vi "Write Filter.vi"(0 "fpga reference in":T2, 2 "enable filter":bool=TRUE, 7 "coefficients":T1, 11 "error in":errorcluster) -> (4 "fpga reference out":T2, 15 "error out":errorcluster)   [LabVIEW 2019]
uses:
  TypeDefs/Blank FPGA Reference.ctl
  <vilib>/rvi/errors/niLvFpgaAdjustHostInterfaceError.vi
  <vilib>/rvi/interface/nirviReadWriteControl/nirviReadWriteControl.xnode
  <vilib>/rvi/interface/Simulation/niFpgaSimulationCallBeginRW.vi
  NiFpgaLv.dll
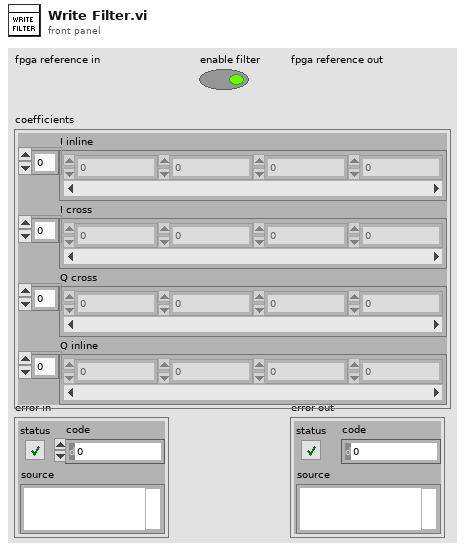
[diagram p1: front panel]
types:
  T1 = cluster{"I inline":dbl[], "I cross":dbl[], "Q cross":dbl[], "Q inline":dbl[]}
  T2 = typedef "Blank FPGA Reference.ctl" = refnum<k20>
  T3 = enum8{"None", "I Inline", "I Cross", "Q Cross", "Q Inline"}
  T4 = cluster{"filter select":enum8{"None", "I Inline", "I Cross", "Q Cross", "Q Inline"}, "coef load":bool, "coef write":bool, "coef data":fxp<+/-,18,1>}
  T5 = enum8{"None", "I Inline", "I Cross", "Q Cross", "Q Inline"}[]
  T6 = cluster{"filter select":enum8{"None", "I Inline", "I Cross", "Q Cross", "Q Inline"}, "coef load":bool, "coef write":bool, "coef data":fxp<+/-,18,1>}[]
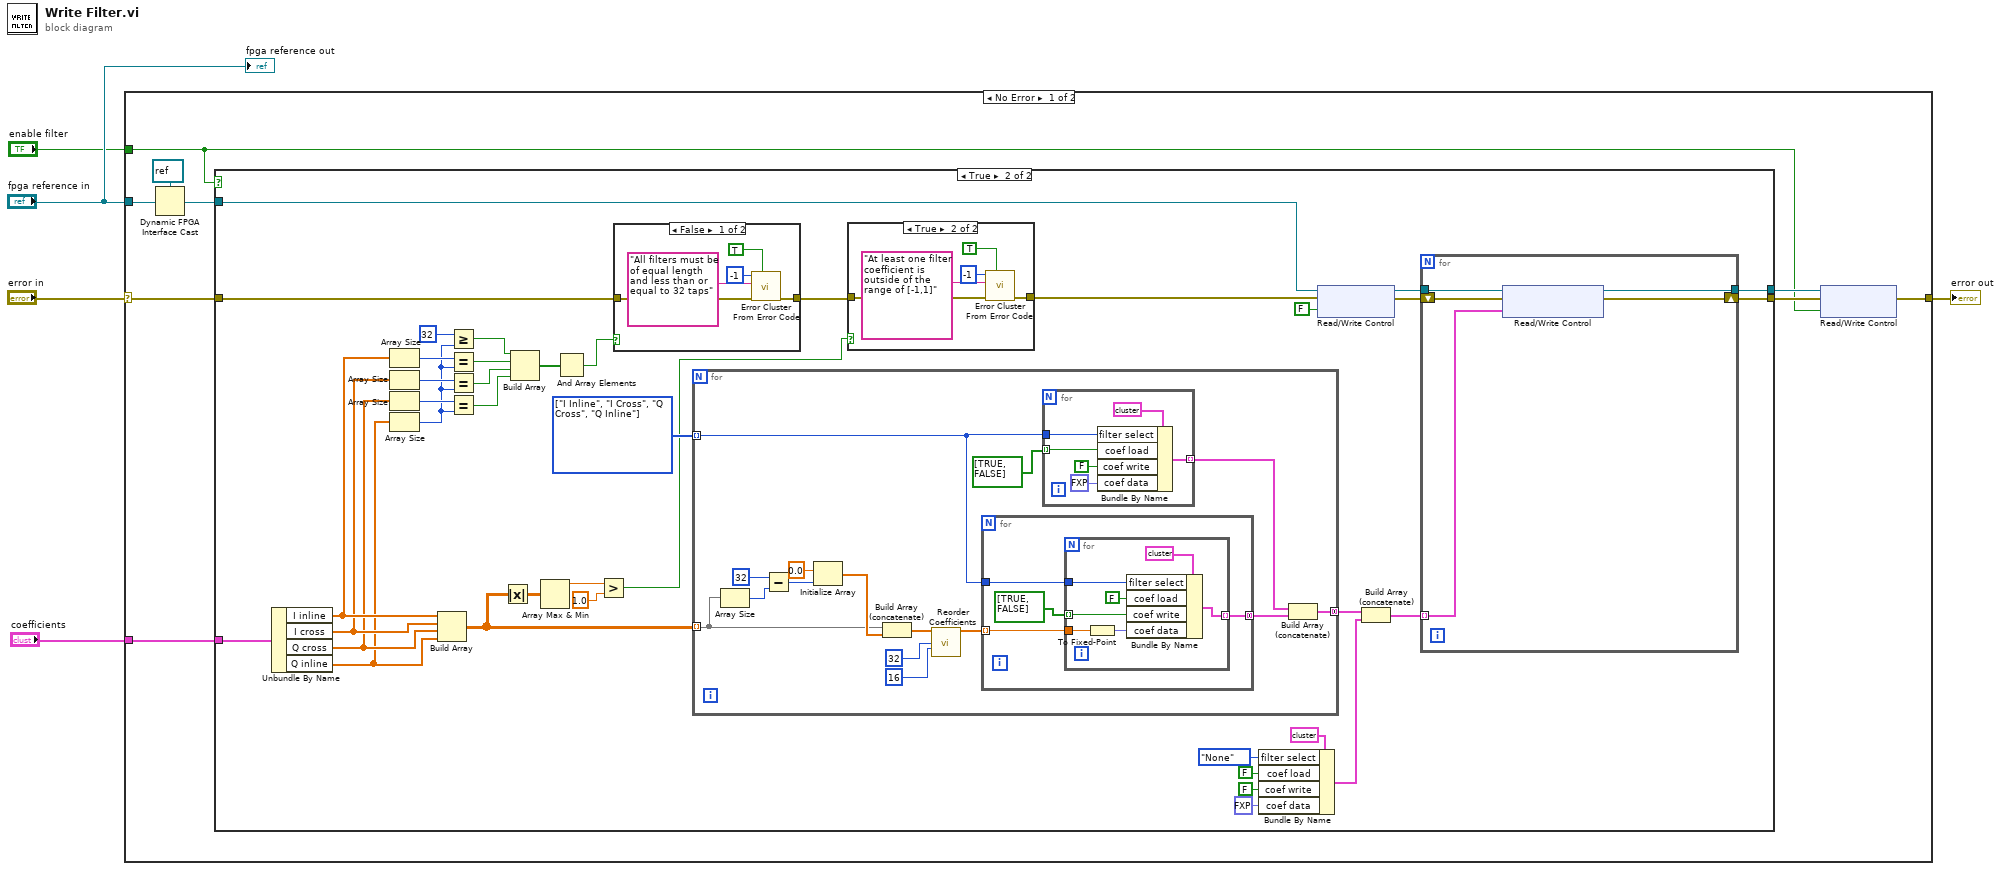
[diagram p0: block diagram]
diagram:
  n1 = case shown="No Error" "error in" {
    selector: "error in" -> [w12 w105]
    tunnel: [w8 w105] -> w5
    tunnel: "fpga reference in" -> [w14 _]
    tunnel: "coefficients" -> [w11 _]
    tunnel: "enable filter" -> [w6 _]
    frame No Error {
      n2 = Dynamic FPGA Interface Cast(Session In=refnum<k20> refnum ("Refnum in"), Type=w14) -> (Session Out=w7:refnum<k20>)
      n3 = case shown="True" w6 {
        tunnel: w12 -> [w16 w47]
        tunnel: w11 -> [_ w45]
        tunnel: [w15 w29] -> w10
        tunnel: [w16 w28] -> w9
        tunnel: w7 -> [w15 w25]
        frame False {
        }
        frame True {
          w46 = T5 [enum."I Inline", enum."I Cross", enum."Q Cross", enum."Q Inline"] items=["None", "I Inline", "I Cross", "Q Cross", "Q Inline"]
          n4 = Unbundle By Name(w45) -> ("I inline"=w44:dbl[], "I cross"=w43:dbl[], "Q cross"=w42:dbl[], "Q inline"=w41:dbl[])
          n5 = Array Size(array=w44) -> (size(s)=w40:i32)
          n6 = Array Size(array=w43) -> (size(s)=w39:i32)
          n7 = Array Size(array=w42) -> (size(s)=w38:i32)
          n8 = Array Size(array=w41) -> (size(s)=w32:i32)
          n9 = Build Array(w44, w43, w42, w41) -> (w23:dbl[][])
          n10 = Greater Or Equal?(x=32, y=w32) -> (x >= y?=w30:bool)
          n11 = Equal?(x=w40, y=w32) -> (x = y?=w37:bool)
          n12 = Equal?(x=w39, y=w32) -> (x = y?=w36:bool)
          n13 = Equal?(x=w38, y=w32) -> (x = y?=w35:bool)
          n14 = Absolute Value(x=w23) -> (abs(x)=w22:dbl[][])
          n15 = Build Array(w30, w37, w36, w35) -> (w34:bool[])
          n16 = Array Max & Min(array=w22) -> (max value=w20:dbl)  [unwired: 3 out]
          n17 = And Array Elements(Boolean array=w34) -> (logical AND=w33:bool)
          n18 = Greater?(x=w20, y=1.0) -> (0:w18:bool)
          n19 = case shown="False" w33 {
            tunnel: w47 -> [w103 w104]
            tunnel: [w102 w104] -> w21
            frame False {
              n20 = call <vilib>:"Error Cluster From Error Code.vi"("show call chain? (False)"=TRUE, "error in (no error)"=w103, "error message (\"\")"="All filters must be of equal length and less than or equal to 32 taps" ("error message (\"\")"), "error code (0)"=-1) -> ("error out"=w102:errorcluster)  [unwired: 5 in]
            }
            frame True {
            }
          }
          n21 = for {
            tunnel: [w69] -> w55 mode=concatenating
            tunnel: w46 -> [w73] mode=indexing
            tunnel: w23 -> [w63] mode=indexing
            n22 = Array Size(array=w63) -> (size(s)=w67:i32)
            n23 = Subtract(x=32, y=w67) -> (x-y=w66:i32)
            n24 = Initialize Array(0.0 ("element"), w66) -> (w64:dbl[])
            n25 = Build Array (concatenate)(w63, w64) -> (w62:dbl[])
            n26 = call "Reorder Coefficients.vi"("coefficients"=w62, "num coefficients"=32 ("order"), "spc"=16) -> ("reordered coefficients"=w74:dbl[])  [unwired: 12 in]
            n27 = for {
              tunnel: [w86] -> w71 mode=concatenating
              tunnel: w74 -> [w85] mode=indexing
              tunnel: w73 -> [w83]
              n28 = for {
                tunnel: [w93] -> w86 mode=indexing
                tunnel: w85 -> [w92]
                tunnel: bool[] [TRUE, FALSE] -> [w90] mode=indexing
                tunnel: w83 -> [w87]
                n29 = To Fixed-Point(number=w92) -> (fixed-point=w91:fxp<+/-,18,1>)  [unwired: 1 in]
                n30 = Bundle By Name(cluster=T4 {"filter select"=enum."None", "coef load"=FALSE, "coef write"=FALSE, "coef data"=0.0} ("filter coefficients"), "filter select"=w87, "coef load"=FALSE ("enable"), "coef write"=w90, "coef data"=w91) -> (w93:T4)
              }
            }
            n31 = for {
              tunnel: w73 -> [w81]
              tunnel: bool[] [TRUE, FALSE] -> [w78] mode=indexing
              tunnel: [w77] -> w70 mode=indexing
              n32 = Bundle By Name(cluster=T4 {"filter select"=enum."None", "coef load"=FALSE, "coef write"=FALSE, "coef data"=0.0} ("filter coefficients"), "filter select"=w81, "coef load"=w78, "coef write"=FALSE, "coef data"=fxp<+/-,18,1> 0.0) -> (w77:T4)
            }
            n33 = Build Array (concatenate)(w70, w71) -> (w69:T6)
          }
          n34 = case shown="True" w18 {
            tunnel: w21 -> [w56 w61]
            tunnel: [w56 w60] -> w17
            frame False {
            }
            frame True {
              n35 = call <vilib>:"Error Cluster From Error Code.vi"("show call chain? (False)"=TRUE, "error in (no error)"=w61, "error message (\"\")"="At least one filter coefficient is outside of the range of [-1,1]" ("error message (\"\")"), "error code (0)"=-1) -> ("error out"=w60:errorcluster)  [unwired: 5 in]
            }
          }
          n36 = Bundle By Name(cluster=T4 {"filter select"=enum."None", "coef load"=FALSE, "coef write"=FALSE, "coef data"=0.0} ("filter coefficients"), "filter select"=T3."None", "coef load"=FALSE ("enable"), "coef write"=FALSE, "coef data"=fxp<+/-,18,1> 0.0) -> (w54:T4)
          n37 = xnode "Read/Write Control"("FPGA VI Reference In"=w25, "error in"=w17, "filter.enable"=FALSE ("enable filter")) -> ("FPGA VI Reference Out"=w24:refnum<k20>, "error out"=w26:errorcluster)
          n38 = Build Array (concatenate)(w55, w54) -> (w50:T6)
          n39 = for {
            tunnel: w24 -> [w97]
            shift-right: [w94] -> w28
            shift-left: w26 -> [w98]
            tunnel: w50 -> [w96] mode=indexing
            tunnel: [w95] -> w29
            n40 = xnode "Read/Write Control"("FPGA VI Reference In"=w97, "error in"=w98, "filter.coefficients"=w96) -> ("FPGA VI Reference Out"=w95:refnum<k20>, "error out"=w94:errorcluster)
          }
        }
      }
      n41 = xnode "Read/Write Control"("FPGA VI Reference In"=w10, "error in"=w9, "filter.enable"=w6) -> ("error out"=w8:errorcluster)  [unwired: 1 out]
    }
    frame Error {
    }
  }
  "error out" <- w5
  "fpga reference out" <- "fpga reference in"
